vi "GUI_DG535_v1.0.0.vi"() -> ()   [LabVIEW 2013]
uses:
  Device Drivers/DG645/subVIs/polarity_TypDEf.ctl
  DelayControl_For Multiple Channels_535.ctl
  Device Drivers/DG535/SubVis/channels_TypDef_DG535.ctl
  GUI_DG645/DelayControl2.ctl
  Device Drivers/DG645/subVIs/saveLocal_TypDef.ctl
  Device Drivers/DG535/SubVis/load_typdef.ctl
  Device Drivers/DG535/SubVis/mode_typDef.ctl
  Device Drivers/DG535/SubVis/trigger_YypDEf_Dg535.ctl
  Device Drivers/DG535/SubVis/TrigSlope_Dg535_TypDEf.ctl
  Device Drivers/DG535/SubVis/Impedance_Dg535_TypDef.ctl
panel:
  in  "time to wait (TCP) 2":i32=10
  in  "plot":bool=TRUE
  out "ratio(h)":bool
  out "fixsize":bool
  in  "shotnumber":i32
  out "error (h)":bool
  out "Device Name (h)":string="TS-dg535-1"
  in  "Main Tap":T1(tab)
  in  "polarity.Channel_D":T2=enum."Positive" caption="Polarity"
  in  "polarity.Channel_C":T2=enum."Positive" caption="Polarity"
  in  "polarity.Channel_B":T2=enum."Positive" caption="Polarity"
  in  "polarity.Channel_A":T2=enum."Positive" caption="Polarity"
  in  "amplitude.Channel_C":dbl=4.0 caption="Amplitude (V)"
  in  "amplitude.Channel_D":dbl=4.0 caption="Amplitude (V)"
  in  "amplitude.Channel_B":dbl=4.0 caption="Amplitude (V)"
  in  "amplitude.Channel_A":dbl=4.0 caption="Amplitude (V)"
  in  "Delay.Channel_t0":T3={"Channel"="T0", "reference"=enum."T0", "delay"=0.0} {"delay" format="%+.12f"}
  in  "Delay.Channel_B":T3={"Channel"="B", "reference"=enum."T0", "delay"=0.001} {"delay" format="%+.12f"}
  in  "amplitude.Channel_t0":dbl=4.0 caption="Amplitude (V)"
  in  "polarity.Channel_t0":T2=enum."Positive" caption="Polarity"
  in  "Delay.Channel_A":T3={"Channel"="A", "reference"=enum."T0", "delay"=0.002} {"delay" format="%+.12f"}
  in  "Delay.Channel_C":T3={"Channel"="C", "reference"=enum."T0", "delay"=0.01} {"delay" format="%+.12f"}
  in  "Delay.Channel_D":T3={"Channel"="D", "reference"=enum."T0", "delay"=0.001} {"delay" format="%+.12f"}
  in  "load.Channel_t0":T6=enum."50 Ohm" caption="Impedance"
  in  "load.Channel_A":T6=enum."50 Ohm" caption="Impedance"
  in  "load.Channel_B":T6=enum."50 Ohm" caption="Impedance"
  in  "load.Channel_C":T6=enum."50 Ohm" caption="Impedance"
  in  "load.Channel_D":T6=enum."50 Ohm" caption="Impedance"
  in  "mode.Channel_t0":T7
  in  "mode.Channel_A":T7
  in  "mode.Channel_B":T7
  in  "mode.Channel_C":T7
  in  "mode.Channel_D":T7
  in  "amplitude.Channel_AB":dbl=4.0 caption="Amplitude (V)"
  in  "load.Channel_AB":T6=enum."50 Ohm" caption="Impedance"
  in  "mode.Channel_AB":T7
  in  "mode.Channel_CD":T7
  in  "load.Channel_CD":T6=enum."50 Ohm" caption="Impedance"
  in  "amplitude.Channel_CD":dbl=4.0 caption="Amplitude (V)"
  out "local Port":u16=65445
  out "port or service name":u16=65444
  out "Remote Host":string="192.168.10.21"
  in  "timeout ms (slow resp)":i32=500
  in  "reset":bool
  out "image con closed":bool
  out "image \nconnection":bool
  out "image con closed 2":bool
  out "All Devices (h)":string[](array[string])=["TestStandDelayBox1", "TS-dg535-1"]
  in  "time to wait (TCP)":i32=10
  out "error out":errorcluster
  out "connections (hidden)":variant[](array[variant])=[variant(refnum<k16> refnum), variant(refnum<k16> refnum)]
  in  "time to wait (main loop)":i32=200
  out "Data String":string="amplitude.Channel_t0,4.000000000000\r\namplitude.Channel_AB,4.000000000000\r\namplitude.Channel_CD,4.000000000000\r\namplitude.Channel_A,4.000000000000\r\namplitude.Channel_B,4.000000000000\r\namplitude.Channel_C,4.000000000000\r\namplitude.Channel_D,4.000000000000\r\npolarity.Channel_t0,Positive\r\npolarity.Channel_A,Positive\r\npolarity.Channel_B,Positive\r\npolarity.Channel_C,Positive\r\npolarity.Channel_D,Positive\r\nload.Channel_t0,50 Ohm\r\nload.Channel_A,50 Ohm\r\nload.Channel_AB,50 Ohm\r\nload.Channel_B,50 Ohm\r\nload.Channel_C,50 Ohm\r\nload.Channel_CD,50 Ohm\r\nload.Channel_D,50 Ohm\r\nmode.Channel_t0,TTL\r\nmode.Channel_A,TTL\r\nmode.Channel_AB,TTL\r\nmode.Channel_B,TTL\r\nmode.Channel_C,TTL\r\nmode.Channel_CD,TTL\r\nmode.Channel_D,TTL\r\nreference.Channel_A,T0\r\ndelay.Channel_A,0.002000000000\r\nreference.Channel_B,T0\r\ndelay.Channel_B,0.001000000000\r\nreference.Channel_C,T0\r\ndelay.Channel_C,0.010000000000\r\nreference.Channel_D,T0\r\ndelay.Channel_D,0.001000000000\r\n"
  in  "send":bool
  in  "Local Saving Path":path
  out "String":string="wait>>Load Local,Save Local,Load File,Save,amplitude.Channel_t0,amplitude.Channel_AB,amplitude.Channel_CD,amplitude.Channel_A,amplitude.Channel_B,amplitude.Channel_C,amplitude.Channel_D,Trigger.ExecuteSingleShot,Trigger.Source,Inhibit,Trigger.Rate,polarity.Channel_t0,polarity.Channel_A,polarity.Channel_B,polarity.Channel_C,polarity.Channel_D,load.Channel_t0,load.Channel_A,load.Channel_AB,load.Channel_B,load.Channel_C,load.Channel_CD,load.Channel_D,mode.Channel_t0,mode.Channel_A,mode.Channel_AB,mode.Channel_B,mode.Channel_C,mode.Channel_CD,mode.Channel_D,"
  in  "trigger.InputImpedance":T8
  in  "trigger.TrigSlope":T9
  in  "trigger.BurstCount":i32
  in  "trigger.ExternalTrigLevel":dbl
  in  "trigger.BurstPeriod":i32
  in  "trigger.InternalTrigRate":dbl
  in  "trigger.TrigSource":T10
  in  "Save Local":T11
  in  "Load Local":T11
  in  "Load File":bool
  in  "Save":bool caption="Save File"
  out "stop":bool
  out "error message":string
  out "Data Connection out":bool=TRUE
  # "A"
  # "B"
  # "C"
  # "D"
  # "T0"
  # "="
  # "="
  # "="
  # "="
  # "="
  # "AB"
  # "CD"
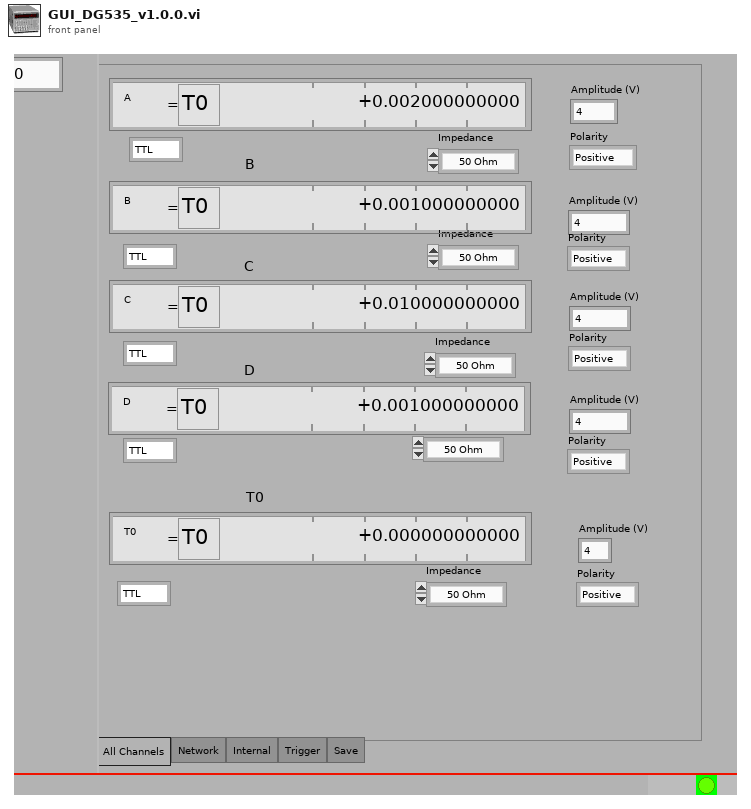
[diagram p1: front panel]
types:
  T1 = enum32{"All Channels", "Network", "Internal", "Trigger", "Save"}
  T2 = typedef "polarity_TypDEf.ctl" = enum16{"Negative", "Positive"}
  T3 = typedef "DelayControl_For Multiple Channels_535.ctl" = cluster{"Channel":string, "reference":T4, "delay":T5}
  T4 = typedef "channels_TypDef_DG535.ctl" = enum16{"T0", "A", "B", "C", "D"}
  T5 = typedef "DelayControl2.ctl" = dbl
  T6 = typedef "load_typdef.ctl" = enum16{"High Z", "50 Ohm"}
  T7 = typedef "mode_typDef.ctl" = enum16{"TTL", "NIM", "ECL", "VAR"}
  T8 = typedef "Impedance_Dg535_TypDef.ctl" = enum16{"High Z", "50 Ohm"}
  T9 = typedef "TrigSlope_Dg535_TypDEf.ctl" = enum16{"-ve edge", "+ve edge"}
  T10 = typedef "trigger_YypDEf_Dg535.ctl" = enum16{"Internal", "External", "Single Shot", "Burst", "Line"}
  T11 = typedef "saveLocal_TypDef.ctl" = enum16{"off", "1", "2", "3", "4", "5", "6", "7", "8", "9"}
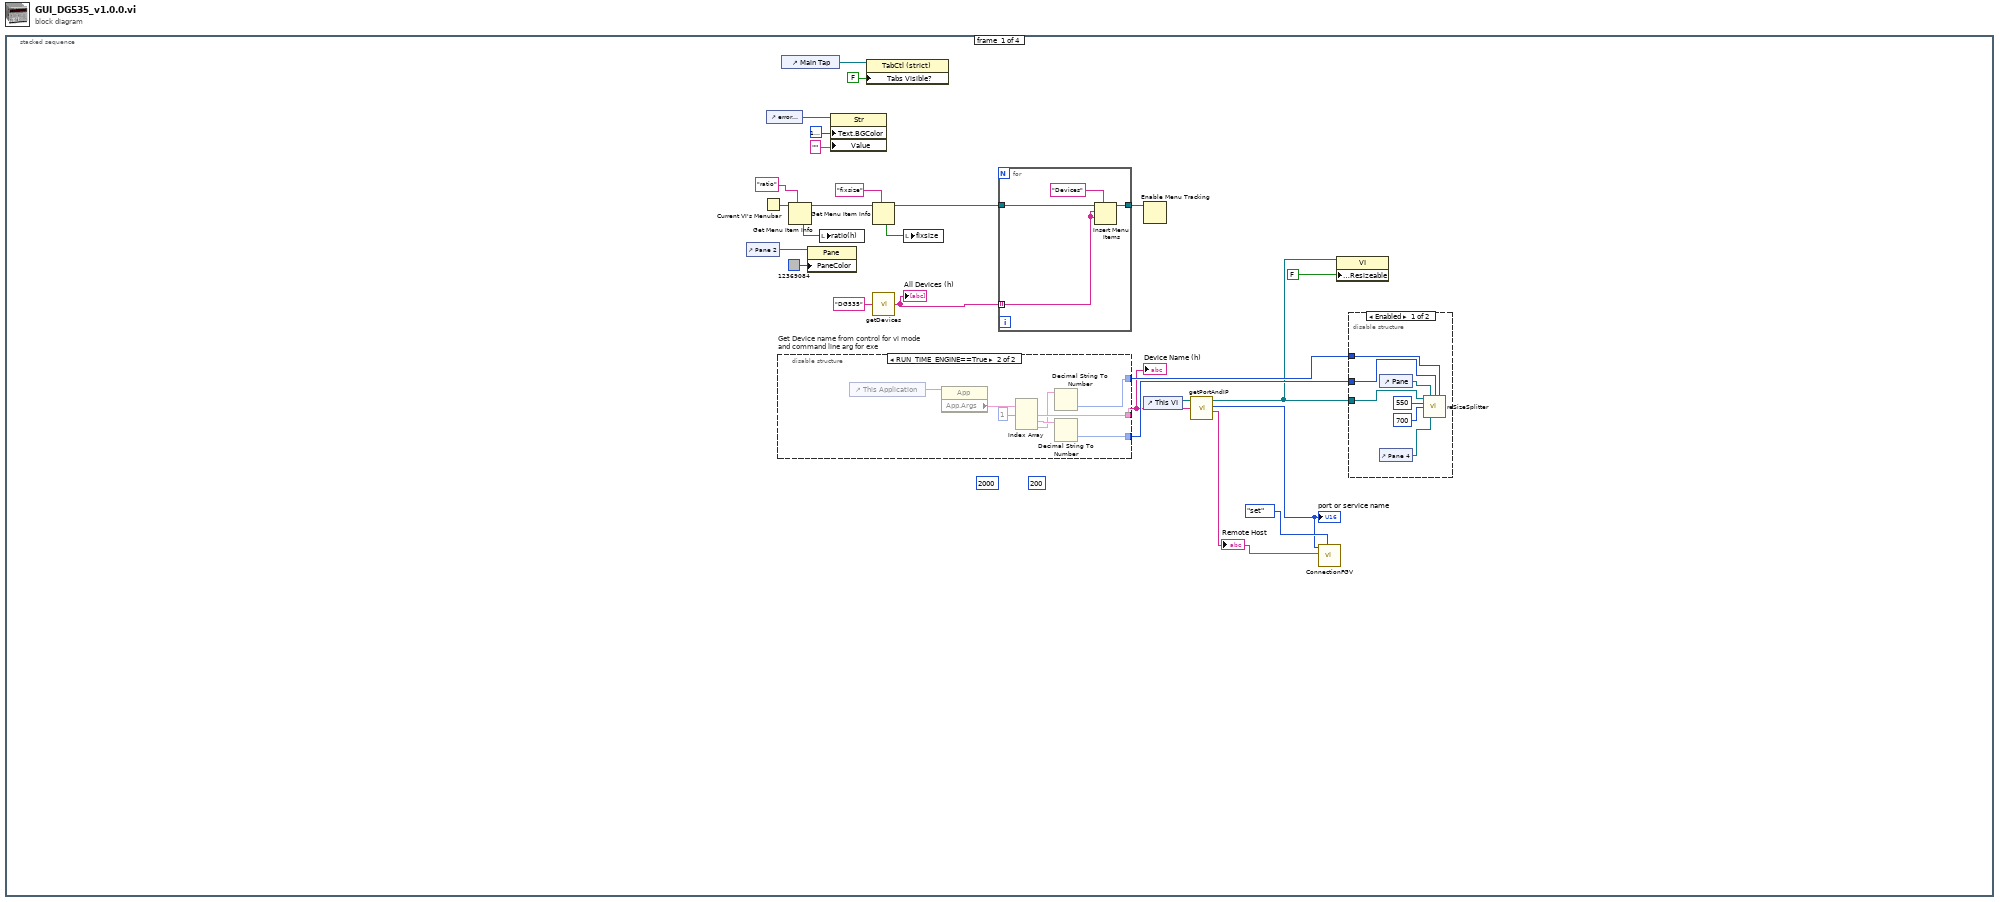
[diagram p0: block diagram]
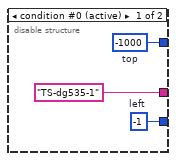
[diagram p3: hidden frame]
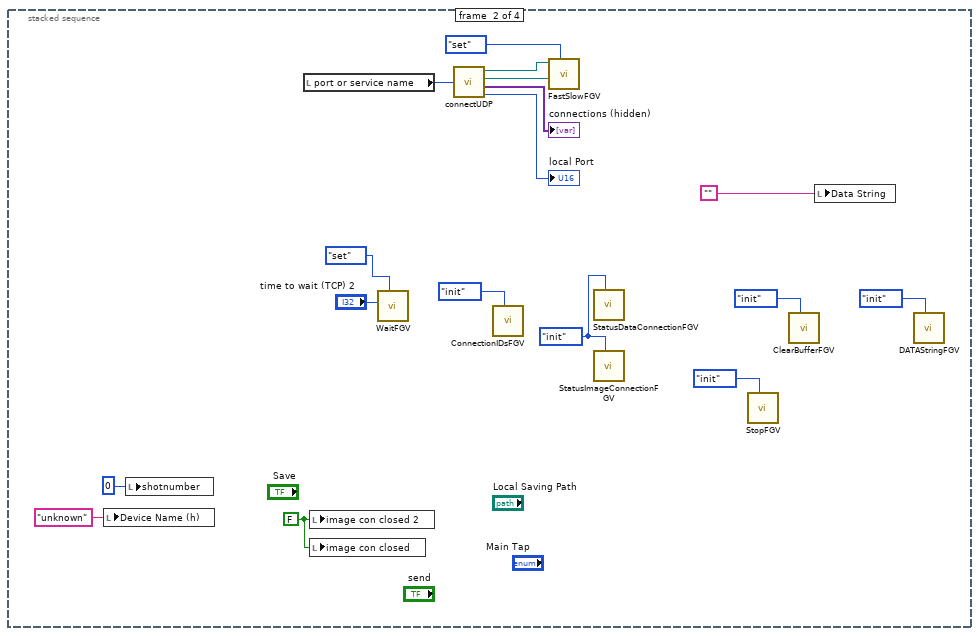
[diagram p4: hidden frame]
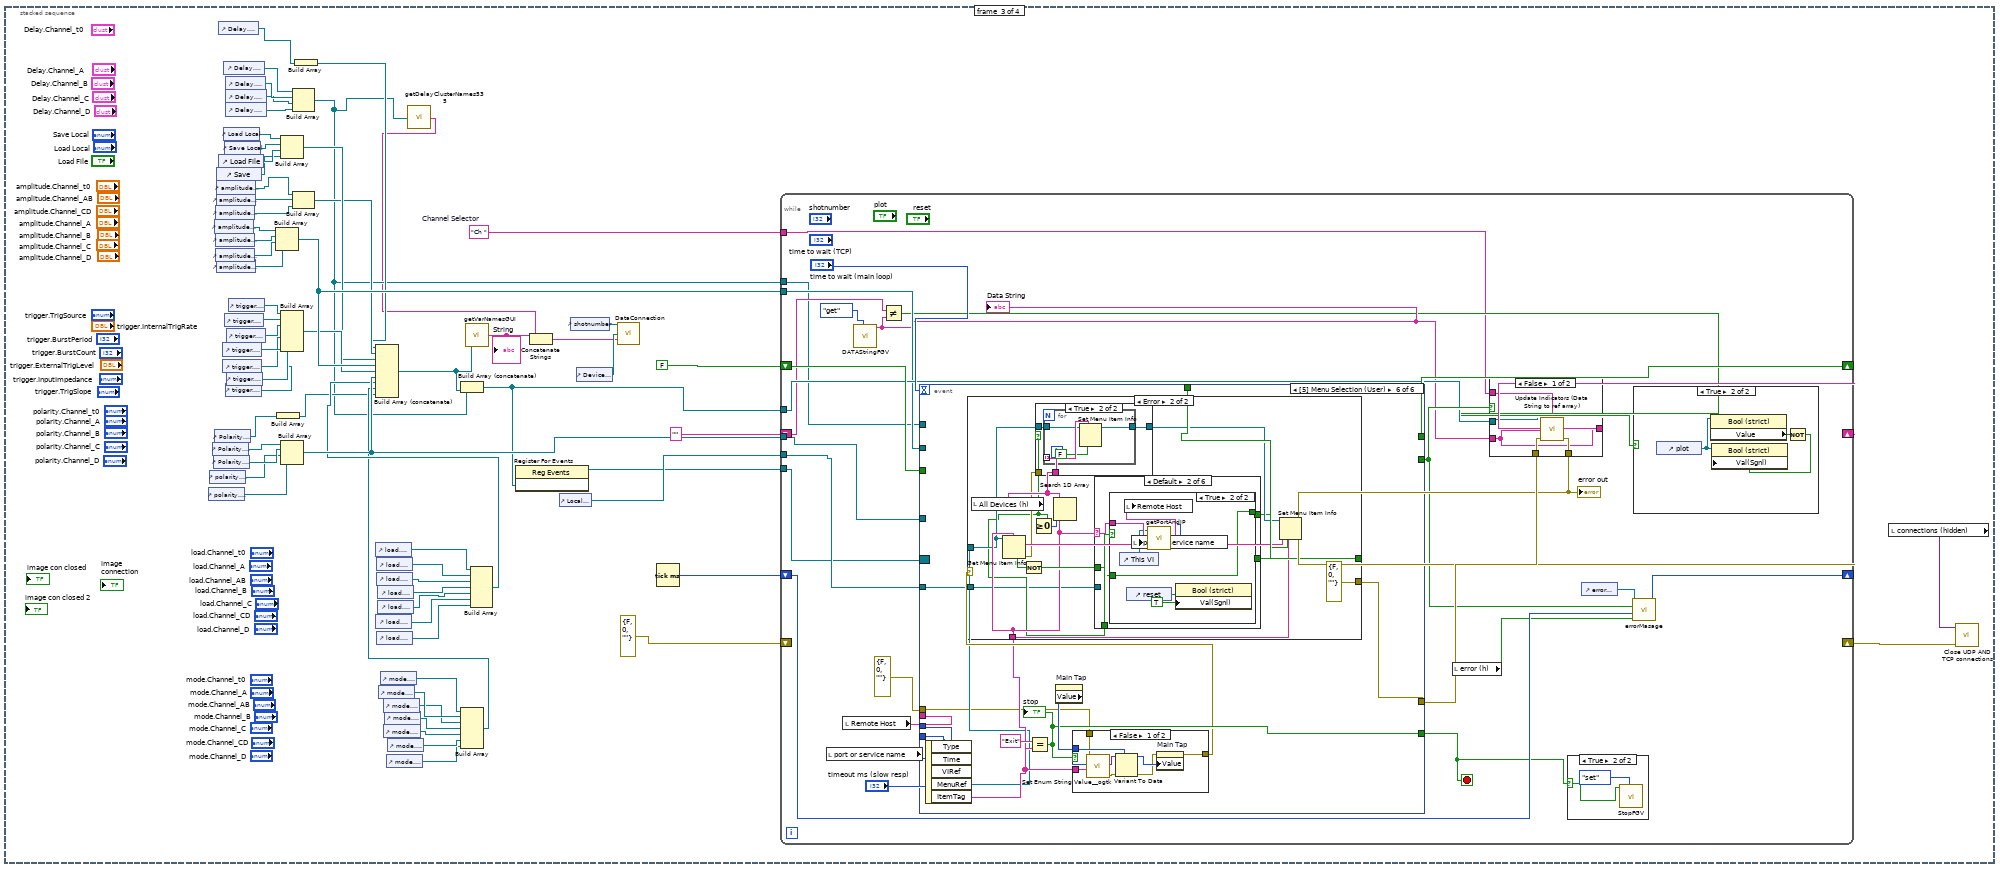
[diagram p5: hidden frame]
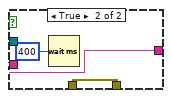
[diagram p8: hidden frame]
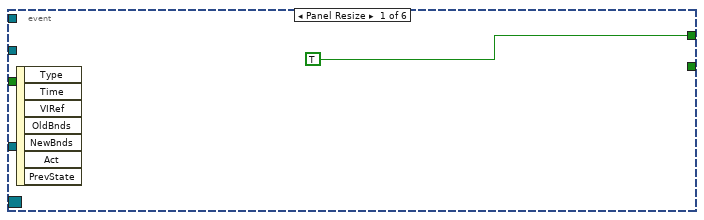
[diagram p9: hidden frame]
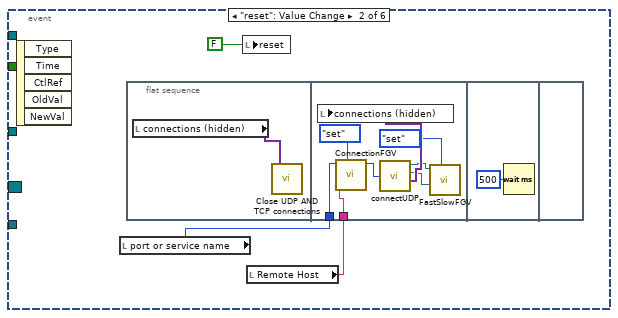
[diagram p10: hidden frame]
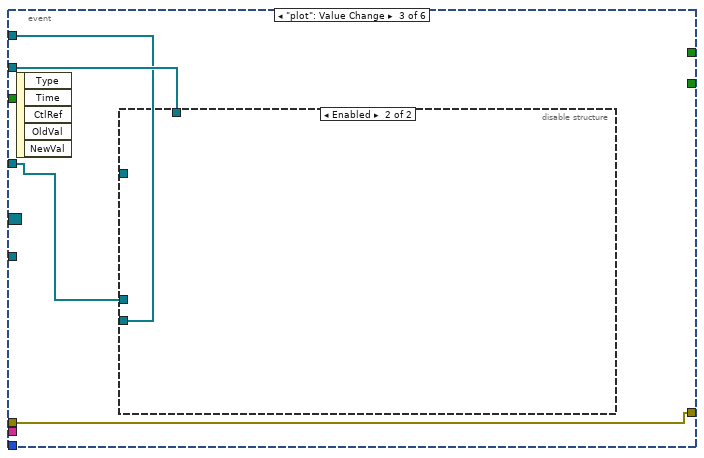
[diagram p11: hidden frame]
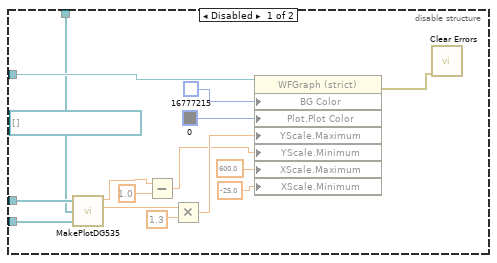
[diagram p12: hidden frame]
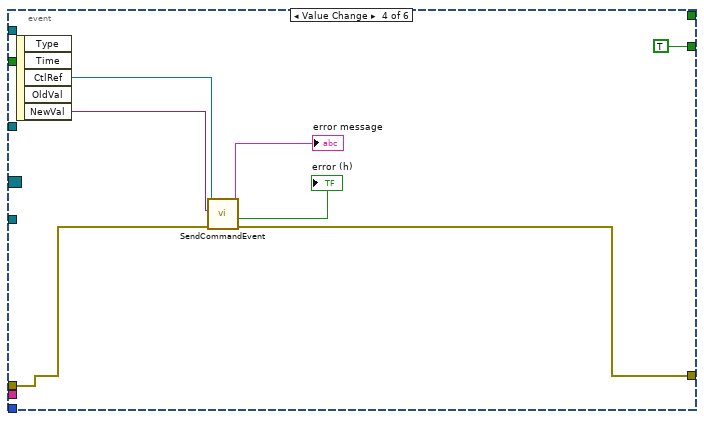
[diagram p13: hidden frame]
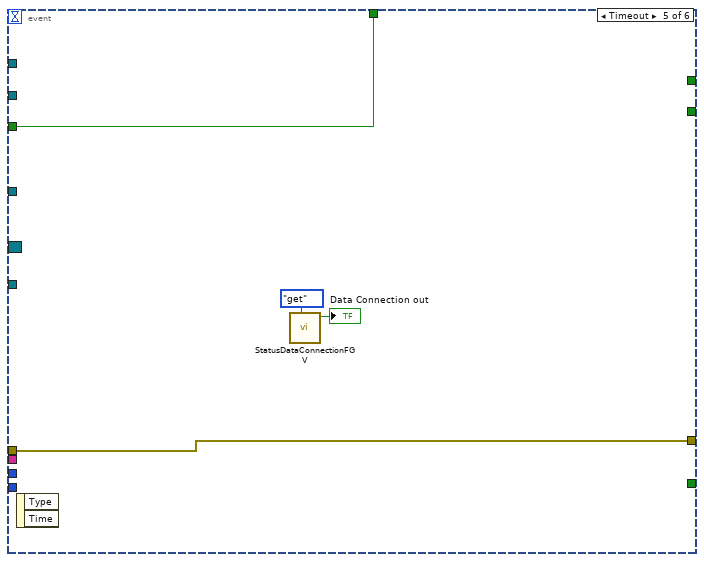
[diagram p14: hidden frame]
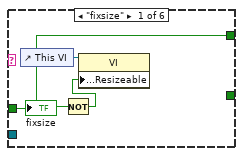
[diagram p17: hidden frame]
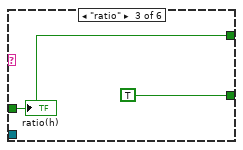
[diagram p19: hidden frame]
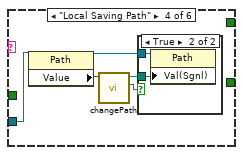
[diagram p20: hidden frame]
diagram:
  n1 = stacked-sequence {
    frame #0 {
      (unwired) i16 2000 ("Left")
      (unwired) i16 200 ("Top")
      n2 = control-ref of="Pane 2"() -> (w13:refnum<vi>)
      n3 = Current VI's Menubar() -> (w23:refnum<k9>)
      n4 = control-ref of="error message"() -> (w15:refnum<vi>)
      n5 = disable-structure "Get Device name from control for vi mode\nand command line arg for exe" shown="RUN_TIME_ENGINE==True" {
        disable-tunnel: ["TS-dg535-1" ("Device Name for vi mode") w45] -> w8
        disable-tunnel: [w39 w42] -> w19
        disable-tunnel: [w38 w41] -> w18
        frame condition #0 (active) {
          w38 = i16 -1000  # top
          w39 = i16 -1  # left
        }
        frame condition #1 {
          n6 = control-ref of="This Application"() -> (w48:refnum<vi>)
          n7 = property class="App"(reference=w48) -> ("App.Args"=w47:string[])  [unwired: 1 in, 2 out]
          n8 = Index Array(array=w47, index #1=1 ("index")) -> (element #1=w45:string, element #2=w44:string, element #3=w43:string)  [unwired: 2 in]
          n9 = Decimal String To Number(string=w43) -> (number=w41:i32)  [unwired: 2 in, 1 out]
          n10 = Decimal String To Number(string=w44) -> (number=w42:i32)  [unwired: 2 in, 1 out]
        }
      }
      "Device Name (h)" <- w8
      n11 = control-ref of="Main Tap"() -> (w26:refnum<vi>)
      n12 = Get Menu Item Info(7:"ratio" ("item tag"), 11:w23) -> (3:w21:refnum<k9>, 4:w22:bool)  [unwired: 1 in, 5 out]
      n13 = property class="Pane"(reference=w13, "PaneColor"=u32 12369084) -> ()  [unwired: 1 in, 2 out]
      n14 = local write "ratio(h)"(w22) -> ()
      n15 = property class="Str"(reference=w15, "Text.BGColor"=u32 16777238, "Value"="") -> ()  [unwired: 1 in, 2 out]
      n16 = property class="TabCtl (strict)"(reference=w26, "Tabs Visible?"=FALSE) -> ()  [unwired: 1 in, 2 out]
      n17 = Get Menu Item Info(7:"fixsize" ("item tag"), 11:w21) -> (3:w11:refnum<k9>, 4:w17:bool)  [unwired: 1 in, 5 out]
      n18 = call "getDevices.vi"("Device Class"="DG535") -> ("All Devices"=w9:string[])
      "All Devices (h)" <- w9
      n19 = local write "fixsize"(w17) -> ()
      n20 = for {
        tunnel: w11 -> [w37]
        tunnel: [w36] -> w10
        tunnel: w9 -> [w34] mode=indexing
        n21 = Insert Menu Items(5:"Devices" ("menu tag"), 7:w34, 8:w34, 9:w37) -> (3:w36:refnum<k9>)  [unwired: 2 in, 2 out]
      }
      n22 = Enable Menu Tracking(4:w10) -> ()  [unwired: 2 in, 2 out]
      n23 = control-ref of="This VI"() -> (w7:refnum<vi>)
      n24 = call "getPortAndIP.vi"("Device Name"=w8, "This Vi"=w7) -> ("Remote Host"=w2:string, "port or service name"=w1:u16, "reference out"=w4:refnum<vi>)  [unwired: 2 in, 2 out]
      "port or service name" <- w1
      "Remote Host" <- w2
      n25 = call "ConnectionFGV.vi"("command"=enum16{"get", "set", "init"}."set", "Remote Host in"=w2, "port or service name in"=w1) -> ()  [unwired: 7 in, 2 out]
      n26 = property class="VI"(reference=w4, "Front Panel.Resizeable"=FALSE ("Front Panel Window:Resizable")) -> ()  [unwired: 1 in, 2 out]
      n27 = disable-structure shown="Enabled" {
        disable-tunnel: w19 -> [w32 _]
        disable-tunnel: w18 -> [w31 _]
        disable-tunnel: w4 -> [w29 _]
        frame Enabled {
          n28 = control-ref of="Pane"() -> (w33:refnum<vi>)
          n29 = control-ref of="Pane 4"() -> (w30:refnum<vi>)
          n30 = call "reSizeSplitter.vi"("this vi"=w29, "pane"=w33, "left"=w32, "top"=w31, "Width"=u32 550, "Height"=u32 700, "pane2"=w30) -> ()  [unwired: 8 in, 1 out]
        }
        frame Disabled {
        }
      }
    }
    frame #1 {
      w57 = enum16{"get", "set", "init"}."init" ("Command")
      w63 = FALSE ("new Device Data")
      n31 = local write "Device Name (h)"("unknown" ("Device Name")) -> ()
      n32 = local write "shotnumber"(0 ("shotnumber")) -> ()
      n33 = local read "port or service name"() -> (w53:u16)
      n34 = local write "image con closed 2"(w63) -> ()
      n35 = local write "image con closed"(w63) -> ()
      n36 = call "WaitFGV.vi"("Command"=enum16{"get", "set", "init"}."set", "milliseconds to wait"="time to wait (TCP) 2") -> ()  [unwired: 9 in, 1 out]
      n37 = call "connectUDP.vi"("port or service name NOT USED"=w53) -> ("fast ID (h)"=w52:refnum<k16>, "slow ID (h)"=w51:refnum<k16>, "connections (hidden)"=→"connections (hidden)":variant[], "local Port"=→"local Port":u16)
      n38 = call "ConnectionIDsFGV.vi"("Command"=enum16{"add", "get", "init"}."init") -> ()  [unwired: 10 in, 1 out]
      n39 = call "FastSlowFGV.vi"("Command"=enum16{"get", "set", "init"}."set", "slow ID"=w51, "fast ID"=w52) -> ()  [unwired: 7 in, 2 out]
      n40 = call "StatusDataConnectionFGV.vi"("Command"=w57) -> ()  [unwired: 10 in, 1 out]
      n41 = call "StatusImageConnectionFGV.vi"("Command"=w57) -> ()  [unwired: 10 in, 1 out]
      n42 = call "StopFGV.vi"("Command"=enum16{"set", "get", "init"}."init") -> ()  [unwired: 9 in, 2 out]
      n43 = call "ClearBufferFGV.vi"("Command"=enum16{"set", "get", "init"}."init") -> ()  [unwired: 10 in, 1 out]
      n44 = local write "Data String"("") -> ()
      n45 = call "DATAStringFGV.vi"("Command"=enum16{"get", "set", "init"}."init") -> ()  [unwired: 9 in, 2 out]
    }
    frame #2 {
      w105 = "Ch "  # Channel Selector
      n46 = control-ref of="polarity.Channel_D"() -> (w99:refnum<vi>)
      n47 = control-ref of="polarity.Channel_C"() -> (w100:refnum<vi>)
      n48 = control-ref of="Polarity.Ch A"() -> (w127:refnum<vi>)
      n49 = control-ref of="Polarity.Ch B"() -> (w126:refnum<vi>)
      n50 = control-ref of="Polarity.Ch T0"() -> (w71:refnum<vi>)
      n51 = control-ref of="amplitude.Channel_A"() -> (w104:refnum<vi>)
      n52 = control-ref of="amplitude.Channel_CD"() -> (w73:refnum<vi>)
      n53 = control-ref of="amplitude.Channel_B"() -> (w103:refnum<vi>)
      n54 = control-ref of="amplitude.Channel_C"() -> (w102:refnum<vi>)
      n55 = control-ref of="Save"() -> (w109:refnum<vi>)
      n56 = control-ref of="amplitude.Channel_AB"() -> (w74:refnum<vi>)
      n57 = control-ref of="amplitude.Channel_D"() -> (w101:refnum<vi>)
      n58 = control-ref of="amplitude.Channel_t0"() -> (w75:refnum<vi>)
      n59 = control-ref of="Delay.Channel_t0"() -> (w69:refnum<vi>)
      n60 = control-ref of="Load File"() -> (w110:refnum<vi>)
      n61 = control-ref of="trigger.BurstCount"() -> (w79:refnum<vi>)
      n62 = control-ref of="trigger.ExternalTrigLevel"() -> (w78:refnum<vi>)
      n63 = control-ref of="Delay.Channel_A"() -> (w125:refnum<vi>)
      n64 = control-ref of="Load Local"() -> (w112:refnum<vi>)
      n65 = control-ref of="Save Local"() -> (w111:refnum<vi>)
      n66 = control-ref of="trigger.InternalTrigRate"() -> (w81:refnum<vi>)
      n67 = control-ref of="Delay.Channel_B"() -> (w124:refnum<vi>)
      n68 = control-ref of="trigger.TrigSlope"() -> (w76:refnum<vi>)
      n69 = control-ref of="Delay.Channel_C"() -> (w123:refnum<vi>)
      n70 = control-ref of="Delay.Channel_D"() -> (w122:refnum<vi>)
      n71 = control-ref of="trigger.BurstPeriod"() -> (w80:refnum<vi>)
      n72 = control-ref of="trigger.InputImpedance"() -> (w77:refnum<vi>)
      n73 = control-ref of="trigger.TrigSource"() -> (w82:refnum<vi>)
      n74 = Build Array(w104, w103, w102, w101) -> (w115:refnum<vi>[])
      n75 = Build Array(w71) -> (w70:refnum<vi>[])
      n76 = Build Array(w127, w126, w100, w99) -> (w114:refnum<vi>[])
      n77 = Build Array(w112, w111, w110, w109) -> (w107:refnum<vi>[])
      n78 = Build Array(w82, w81, w80, w79, w78, w77, w76) -> (w113:refnum<vi>[])
      n79 = Build Array(w125, w124, w123, w122) -> (w67:refnum<vi>[])
      n80 = Build Array(w75, w74, w73) -> (w72:refnum<vi>[])
      n81 = Build Array(w69) -> (w68:refnum<vi>[])
      n82 = control-ref of="load.Channel_t0"() -> (w98:refnum<vi>)
      n83 = control-ref of="load.Channel_CD"() -> (w93:refnum<vi>)
      n84 = control-ref of="load.Channel_A"() -> (w97:refnum<vi>)
      n85 = control-ref of="load.Channel_AB"() -> (w96:refnum<vi>)
      n86 = control-ref of="load.Channel_D"() -> (w92:refnum<vi>)
      n87 = control-ref of="load.Channel_B"() -> (w95:refnum<vi>)
      n88 = control-ref of="load.Channel_C"() -> (w94:refnum<vi>)
      n89 = control-ref of="mode.Channel_A"() -> (w89:refnum<vi>)
      n90 = control-ref of="mode.Channel_t0"() -> (w90:refnum<vi>)
      n91 = control-ref of="mode.Channel_AB"() -> (w88:refnum<vi>)
      n92 = control-ref of="mode.Channel_C"() -> (w86:refnum<vi>)
      n93 = control-ref of="mode.Channel_B"() -> (w87:refnum<vi>)
      n94 = control-ref of="mode.Channel_D"() -> (w84:refnum<vi>)
      n95 = control-ref of="mode.Channel_CD"() -> (w85:refnum<vi>)
      n96 = call "getDelayClusterNames535.vi"("appended array 2"=w67) -> ("spreadsheet string"=w66:string)
      n97 = Build Array(w90, w89, w88, w87, w86, w85, w84) -> (w83:refnum<vi>[])
      n98 = Build Array(w98, w97, w96, w95, w94, w93, w92) -> (w91:refnum<vi>[])
      n99 = Build Array (concatenate)(w68, w72, w107, w115, w113, w114, w91, w83, w70) -> (w108:refnum<vi>[])
      n100 = Build Array (concatenate)(w67, w108) -> (w106:refnum<vi>[])
      n101 = call "getVarNamesGUI.vi"("Array"=w108) -> ("String"=w118:string)  [unwired: 1 in]
      "String" <- w118
      n102 = register-events(w106) -> (reference out=w116:refnum<event-registration>)  [unwired: 2 in, 1 out]
      n103 = Concatenate Strings(w118, w66) -> (w117:string)
      n104 = control-ref of="Local Saving Path"() -> (w128:refnum<vi>)
      n105 = control-ref of="shotnumber"() -> (w120:refnum<vi>)
      n106 = control-ref of="Device Name (h)"() -> (w119:refnum<vi>)
      n107 = call "DataConnection.vi"("Subscriber list"=w117, "Device Name (h)"=w119, "shotnumber"=w120) -> ()
      n108 = Tick Count (ms)() -> (millisecond timer value=w129:u32)
      n109 = while {
        shift-right: [w155] -> w132
        shift-left: errorcluster {"status"=FALSE, "code"=0, "source"=""} ("error out") -> [_]
        tunnel: w106 -> [w147]
        shift-right: [w153] -> _
        shift-left: FALSE -> [w154]
        shift-right: [w152] -> _
        shift-left: w129 -> [w151]
        tunnel: w128 -> [w148]
        tunnel: w114 -> [w146]
        tunnel: w115 -> [w145]
        tunnel: w67 -> [w137]
        shift-right: [w144] -> _
        shift-left: "" ("Data String") -> [w142]
        tunnel: w116 -> [w138]
        tunnel: w105 -> [w135]
        stop <- w139 stop-if-true
        n110 = local read "port or service name"() -> (w157:u16)
        n111 = local read "Remote Host"() -> (w158:string)
        n112 = call "DATAStringFGV.vi"("Command"=enum16{"get", "set", "init"}."get") -> ("Data String out"=w141:string)  [unwired: 9 in, 1 out]
        "Data String" <- w141
        n113 = Not Equal?(x=w142, y=w141) -> (x != y?=w140:bool)
        n114 = event shown="[5] Menu Selection (User)" {
          selector: w138 -> [_ _ _ _ _ _]
          dyn-events: _ -> [_ _ _ _ _ _]
          timeout: "time to wait (main loop)" -> [_ _ _ _ _ _]
          tunnel: [_ _ w188 w212 w218 w219] -> w156
          tunnel: w158 -> [_ _ _ _ _ _]
          tunnel: w157 -> [_ _ _ _ _ _]
          tunnel: "timeout ms (slow resp)" -> [_ _ _ _ _ _]
          tunnel: errorcluster {"status"=FALSE, "code"=0, "source"=""} ("error out") -> [_ _ w188 w208 w218 w220]
          tunnel: [_ _ _ TRUE _ _] -> w149
          tunnel: [_ _ _ _ _ w226] -> w139
          tunnel: [_ _ _ _ w217 w223] -> _
          tunnel: w154 -> [_ _ _ _ w217 _]
          tunnel: [TRUE _ _ _ _ _] -> w153
          tunnel: w148 -> [_ _ _ _ _ w221]
          tunnel: w146 -> [_ _ w191 _ _ _]
          tunnel: w145 -> [_ _ w190 _ _ _]
          tunnel: w137 -> [_ _ w189 _ _ _]
          event Panel Resize {
            n115 = event-data() -> ()  [unwired: 1 in, 7 out]
          }
          event "reset": Value Change {
            n116 = event-data() -> ()  [unwired: 1 in, 5 out]
            n117 = local read "port or service name"() -> (w176:u16)
            n118 = flat-sequence {
              tunnel: w176 -> [w181]
              tunnel: w175 -> [w180]
              frame #0 {
                n119 = local read "connections (hidden)"() -> (w178:variant[])
                n120 = call "Close UDP AND TCP connections.vi"("appended array"=w178) -> ()  [unwired: 7 in]
              }
              frame #1 {
                n121 = call "ConnectionFGV.vi"("command"=enum16{"get", "set", "init"}."set", "Remote Host in"=w180, "port or service name in"=w181) -> ("port or service name out"=w185:u16)  [unwired: 7 in, 1 out]
                n122 = call "connectUDP.vi"("port or service name NOT USED"=w185) -> ("fast ID (h)"=w183:refnum<k16>, "slow ID (h)"=w182:refnum<k16>, "connections (hidden)"=w184:variant[])  [unwired: 1 out]
                n123 = local write "connections (hidden)"(w184) -> ()
                n124 = call "FastSlowFGV.vi"("Command"=enum16{"get", "set", "init"}."set", "slow ID"=w182, "fast ID"=w183) -> ()  [unwired: 7 in, 2 out]
              }
              frame #2 {
                n125 = Wait (ms)(milliseconds to wait=u32 500) -> ()  [unwired: 1 out]
              }
              frame #3 {
              }
            }
            n126 = local write "reset"(FALSE ("reset")) -> ()
            n127 = local read "Remote Host"() -> (w175:string)
          }
          event "plot": Value Change {
            n128 = event-data() -> ()  [unwired: 1 in, 5 out]
            n129 = disable-structure shown="Enabled" {
              disable-tunnel: _ -> [w199 _]
              disable-tunnel: w191 -> [w198 _]
              disable-tunnel: w190 -> [w197 _]
              disable-tunnel: w189 -> [w192 _]
              frame Disabled {
                (unwired) refnum<vi>[] [] ("Channel array")
                n130 = call "MakePlotDG535.vi"("Polarity array"=w198, "Amplitude array"=w197, "Channel array"=w192) -> ("min value"=w194:dbl, "Numeric 3"=w203:dbl, "Array"=w200:cluster{"Pulse Pattern":dbl[]}[])  [unwired: 2 out]
                n131 = Subtract(x=w194, y=1.0) -> (x-y=w193:dbl)
                n132 = Multiply(x=w203, y=1.3) -> (x*y=w205:dbl)
                n133 = property class="WFGraph (strict)"(reference=w199, "BG Color"=u32 16777215 ("Color"), "Plot.Plot Color"=u32 0 ("Color"), "YScale.Maximum"=w205, "YScale.Minimum"=w193, "XScale.Maximum"=600.0 ("X Scale.Range:Maximum"), "XScale.Minimum"=-25.0 ("X Scale.Range:Minimum")) -> (error out=w195:errorcluster)  [unwired: 1 in, 1 out]
                n134 = call <vilib>:"Clear Errors.vi"("error in (no error)"=w195) -> ()  [unwired: 6 in, 1 out]
              }
              frame Enabled {
              }
            }
          }
          event Value Change {
            n135 = event-data() -> ("CtlRef"=w214:refnum<vi>, "NewVal"=w213:variant)  [unwired: 1 in, 3 out]
            n136 = call "SendCommandEvent.vi"("error out 2"=w208, "NewVal"=w213, "CtlRef"=w214) -> ("error out"=w212:errorcluster, "error (h)"=→"error (h)":bool, "error message"=→"error message":string)  [unwired: 5 in, 1 out]
          }
          event Timeout {
            n137 = event-data() -> ()  [unwired: 1 in, 2 out]
            n138 = call "StatusDataConnectionFGV.vi"("Command"=enum16{"get", "set", "init"}."get") -> ("Data Connection out"=→"Data Connection out":bool)  [unwired: 10 in]
          }
          event Menu Selection (User) {
            n139 = event-data() -> ("MenuRef"=w222:refnum<k9>, "ItemTag"=w224:string)  [unwired: 1 in, 3 out]
            n140 = Equal?(x="Exit", y=w224) -> (x = y?=w226:bool)
            "stop" <- w226
            n141 = property on="Main Tap" class="TabCtl (strict)"() -> ("Value"=w228:T1)  [unwired: 2 in, 2 out]
            n142 = case shown="False" w226 {
              tunnel: w228 -> [w284 _]
              tunnel: w224 -> [w283 _]
              tunnel: [w280 errorcluster {"status"=FALSE, "code"=0, "source"=""} ("error out")] -> w225
              tunnel: w220 -> [w279 _]
              frame False {
                n143 = call <userlib>:"Set Enum String Value__ogtk.vi"("error in (no error)"=w279, "String Value"=w283, "Default Enum Value"=w284) -> ("error out"=w282:errorcluster, "Enum"=w286:variant)  [unwired: 7 in]
                n144 = Variant To Data(error in=w282, type=w284, Variant=w286) -> (data=w285:T1, error out=w281:errorcluster)
                n145 = property on="Main Tap" class="TabCtl (strict)"(error in=w281, "Value"=w285) -> (error out=w280:errorcluster)  [unwired: 1 in, 1 out]
              }
              frame True {
              }
            }
            n146 = case shown="Error" w225 {
              selector: w225 -> [w229 _]
              tunnel: w222 -> [_ w235]
              tunnel: w224 -> [_ w239]
              tunnel: [_ w240] -> w223
              tunnel: w221 -> [_ w233]
              tunnel: [w229 errorcluster {"status"=FALSE, "code"=0, "source"=""} ("error IO")] -> w219
              frame No Error {
              }
              frame Error {
                n147 = local read "All Devices (h)"() -> (w237:string[])
                n148 = Get Menu Item Info(7:w239, 11:w235) -> (0:w236:errorcluster, 2:w242:string, 4:w243:bool)  [unwired: 1 in, 4 out]
                n149 = Not(x=w243) -> (.not. x?=w241:bool)
                n150 = Search 1D Array(1D array=w237, element=w239) -> (index of element=w238:i32)  [unwired: 1 in]
                n151 = Greater Or Equal To 0?(x=w238) -> (x >= 0?=w234:bool)
                n152 = case shown="True" w234 {
                  tunnel: w237 -> [_ w247]
                  tunnel: w236 -> [_ _]
                  tunnel: w235 -> [w244 w246]
                  tunnel: [w244 w245] -> w232
                  frame False {
                  }
                  frame True {
                    n153 = for {
                      tunnel: w247 -> [w251] mode=indexing
                      tunnel: w246 -> [w249]
                      tunnel: [w248] -> w245
                      n154 = Set Menu Item Info(6:FALSE ("checked"), 7:w251, 11:w249) -> (3:w248:refnum<k9>)  [unwired: 4 in, 1 out]
                    }
                  }
                }
                n155 = case shown="Default" w239 {
                  selector: w239 -> [_ w257 _ _ _ _]
                  tunnel: w241 -> [w252 w255 w266 _ _ _]
                  tunnel: [_ _ TRUE _ _ _] -> w240
                  tunnel: w234 -> [_ w258 _ _ _ _]
                  tunnel: w233 -> [_ _ _ w272 _ _]
                  tunnel: [w252 w256 w266 _ _ _] -> w231
                  frame "fixsize" {
                    n156 = control-ref of="This VI"() -> (w254:refnum<vi>)
                    n157 = Not(x=w252) -> (.not. x?=w253:bool)
                    n158 = property class="VI"(reference=w254, "Front Panel.Resizeable"=w253) -> ()  [unwired: 1 in, 2 out]
                    "fixsize" <- w252
                  }
                  frame Default {
                    n159 = case shown="True" w258 {
                      tunnel: w257 -> [_ w265]
                      tunnel: [_ w259] -> w256
                      tunnel: w255 -> [_ w259]
                      frame False {
                      }
                      frame True {
                        n160 = control-ref of="This VI"() -> (w264:refnum<vi>)
                        n161 = control-ref of="reset"() -> (w261:refnum<vi>)
                        n162 = call "getPortAndIP.vi"("Device Name"=w265, "This Vi"=w264) -> ("Remote Host"=w263:string, "port or service name"=w262:u16)  [unwired: 2 in, 3 out]
                        n163 = local write "Remote Host"(w263) -> ()
                        n164 = local write "port or service name"(w262) -> ()
                        n165 = property class="Bool (strict)"(reference=w261, "Val(Sgnl)"=TRUE ("Value (Signaling)")) -> ()  [unwired: 1 in, 2 out]
                      }
                    }
                  }
                  frame "ratio" {
                    "ratio(h)" <- w266
                  }
                  frame "Local Saving Path" {
                    n166 = property class="Path"(reference=w272) -> (reference out=w270:refnum<vi>, "Value"=w271:path)  [unwired: 1 in, 1 out]
                    n167 = call "changePath.vi"("Local Saving in (h)"=w271) -> ("change (h)"=w269:bool, "Local Saving out (h)"=w268:path)  [unwired: 9 in]
                    n168 = case shown="True" w269 {
                      tunnel: w270 -> [_ w274]
                      tunnel: w268 -> [_ w273]
                      frame False {
                      }
                      frame True {
                        n169 = property class="Path"(reference=w274, "Val(Sgnl)"=w273) -> ()  [unwired: 1 in, 2 out]
                      }
                    }
                  }
                  frame "reset" {
                    n170 = control-ref of="reset"() -> (w276:refnum<vi>)
                    n171 = property class="Bool (strict)"(reference=w276, "Val(Sgnl)"=TRUE ("Value (Signaling)")) -> ()  [unwired: 1 in, 2 out]
                  }
                  frame "clear" {
                    n172 = control-ref of="reset"() -> (w278:refnum<vi>)
                    n173 = property class="Bool (strict)"(reference=w278, "Val(Sgnl)"=TRUE ("Value (Signaling)")) -> ()  [unwired: 1 in, 2 out]
                  }
                }
                n174 = Set Menu Item Info(6:w231, 7:w239, 10:w242, 11:w232) -> ()  [unwired: 3 in, 2 out]
              }
            }
          }
        }
        n175 = local read "error (h)"() -> (w136:bool)
        n176 = case shown="False" w149 {
          tunnel: w147 -> [w169 _]
          tunnel: w156 -> [w168 w173]
          tunnel: [w170 w173] -> w155
          tunnel: w135 -> [w166 _]
          tunnel: [w167 w171] -> w144
          tunnel: w141 -> [w167 w171]
          frame False {
            n177 = call "Update Indicators (Data String to ref array).vi"("Array"=w169, "Active Channel"=w166, "Data String"=w167, "error in (no error)"=w168) -> ("error out"=w170:errorcluster)  [unwired: 10 in, 1 out]
          }
          frame True {
            n178 = Wait (ms)(milliseconds to wait=u32 400) -> ()  [unwired: 1 out]
          }
        }
        "error out" <- w155
        n179 = case shown="True" w139 {
          selector: w139 -> [_ w161]
          frame False {
          }
          frame True {
            n180 = call "StopFGV.vi"("Command"=enum16{"set", "get", "init"}."set", "Stop"=w161) -> ()  [unwired: 8 in, 2 out]
          }
        }
        n181 = control-ref of="error message"() -> (w150:refnum<vi>)
        n182 = call "errorMasage.vi"("error (h)"=w136, "millisecond timer value"=w151, "Boolean"=w149, "error message"=w150) -> ("millisecond timer value 2"=w152:u32)
        n183 = case shown="True" w140 {
          frame False {
          }
          frame True {
            n184 = control-ref of="plot"() -> (w165:refnum<vi>)
            n185 = property class="Bool (strict)"(reference=w165) -> ("Value"=w164:bool)  [unwired: 1 in, 2 out]
            n186 = Not(x=w164) -> (.not. x?=w163:bool)
            n187 = property class="Bool (strict)"(reference=w165, "Val(Sgnl)"=w163) -> ()  [unwired: 1 in, 2 out]
          }
        }
      }
      n188 = local read "connections (hidden)"() -> (w131:variant[])
      n189 = call "Close UDP AND TCP connections.vi"("error in"=w132, "appended array"=w131) -> ()  [unwired: 6 in]
    }
    frame #3 {
      n190 = flat-sequence {
        frame #0 {
          n191 = Wait (ms)(milliseconds to wait=u32 0) -> ()  [unwired: 1 out]
        }
        frame #1 {
          n192 = local write "stop"(FALSE ("stop")) -> ()
        }
        frame #2 {
          n193 = control-ref of="This VI"() -> (w295:refnum<vi>)
          n194 = case shown="True" FALSE {
            tunnel: w295 -> [w296 w299]
            tunnel: [w296 w297] -> w294
            frame False {
            }
            frame True {
              n195 = property class="VI" props=["Front Panel.Open"](reference=w299) -> (reference out=w298:refnum<vi>)  [unwired: 1 in, 2 out]
              n196 = invoke class="VI" method="FP.Close"(reference=w298) -> (reference out=w297:refnum<vi>)  [unwired: 2 in, 2 out]
            }
          }
          n197 = Close Reference(reference=w294) -> ()  [unwired: 1 in, 1 out]
        }
      }
      n198 = control-ref of="Main  Control"() -> (w289:refnum<vi>)
      n199 = property class="TabCtl (strict)"(reference=w289, "Tabs Visible?"=TRUE) -> ()  [unwired: 1 in, 2 out]
      n200 = property class="TabCtl (strict)"(reference=w289, "Tab Location"=enum32{"Top", "Bottom", "Left", "Right"}."Bottom") -> ()  [unwired: 1 in, 2 out]
    }
  }
